vi "CFG Read_Write File.vi"(0 "Cluster In Ref":refnum<vi>, 1 "System Configuration File":path=path "inifiles/System Configuration.ini", 2 "Array In":T1[](array[typedef]), 5 "Cluster Out Ref":refnum<vi>, 7 "Enum Ref":refnum<vi>, 11 "Error In (no error)":errorcluster, 12 "Keys (Empty:All)":string[](array[string]), 13 "Operation":T5) -> (4 "Array":T1[](array[typedef]), 15 "Error Out":errorcluster)   [LabVIEW 2012]
uses:
  Type Defs/CFG File Operation Enum.ctl
  Type Defs/CFG Key Cluster.ctl
  Type Defs/CFG Tag Type Enum.ctl
  <vilib>/Utility/config.llb/Read Key (Boolean).vi
  <vilib>/Utility/config.llb/Read Key (String).vi
  <vilib>/Utility/config.llb/Read Key (Path).vi
  <vilib>/Utility/config.llb/Write Key (String).vi
  <vilib>/Utility/config.llb/Write Key (Boolean).vi
  <vilib>/Utility/config.llb/Write Key (Path).vi
  <vilib>/Utility/config.llb/NI_LVConfig.lvlib
panel:
  in  "Test Enum":T3(ring)
  in  "Test System In":T4 {"Settings"."Frequency" format="%_4p Hz"; "Settings"."Power" format="%.3f"; "Settings"."Code" format="%.0x"}
  out "Test System Out":T4 {"Settings"."Frequency" format="%_4p Hz"; "Settings"."Power" format="%.3f"; "Settings"."Code" format="%.0x"}
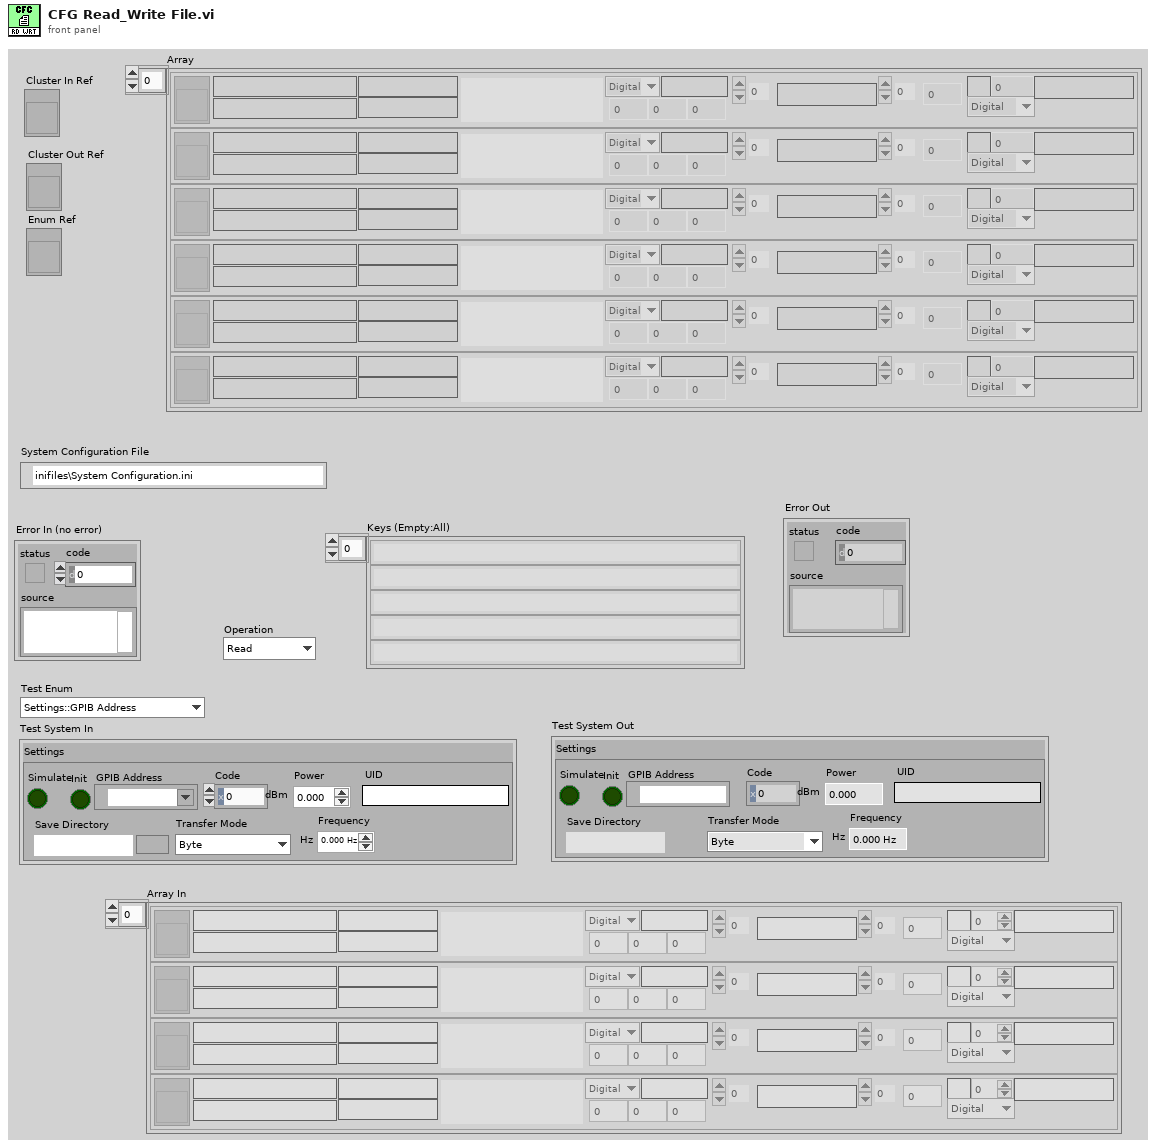
[diagram p1: front panel]
types:
  T1 = typedef "CFG Key Cluster.ctl" = cluster{"Strings []":string[], "Disabled Items []":i32[], "Value":variant, "Format String":string, "Tag":string, "Type":T2, "Section":string, " Ctl Ref":refnum<vi>, "Data Range":cluster{"Minimum":dbl, "Maximum":dbl, "Increment":dbl}, "Unit":string, "Special Instructions":string, "Delimiter(s)":string, "Dimensions":i32, "Element Type":T2, "Array Value String":string}
  T2 = typedef "CFG Tag Type Enum.ctl" = enum16{"Digital", "Slide", "Enum", "Boolean", "String", "Path", "Array", "VISAResourceName", "DAQmxName", "Cluster"}
  T3 = enum16{"Settings::GPIB Address", "Settings::Simulate", "Settings::Code", "Settings::Power", "Settings::UID", "Settings::Save Directory", "Settings::Transfer Mode", "Settings::Frequency"}
  T4 = cluster{"Settings":cluster{"Simulate":bool, "Init":bool, "GPIB Address":refnum<visa-resource-name>, "Save Directory":path, "Transfer Mode":enum16{"Byte", "Word", "LongWord"}, "Code":u8, "Power":dbl, "Frequency":dbl, "UID":string}}
  T5 = typedef "CFG File Operation Enum.ctl" = enum16{"Read", "Write", "Copy", "Edit"}
  T6 = typedef "NI_LVConfig.lvlib/Config Data RefNum.ctl" = refnum<k1>
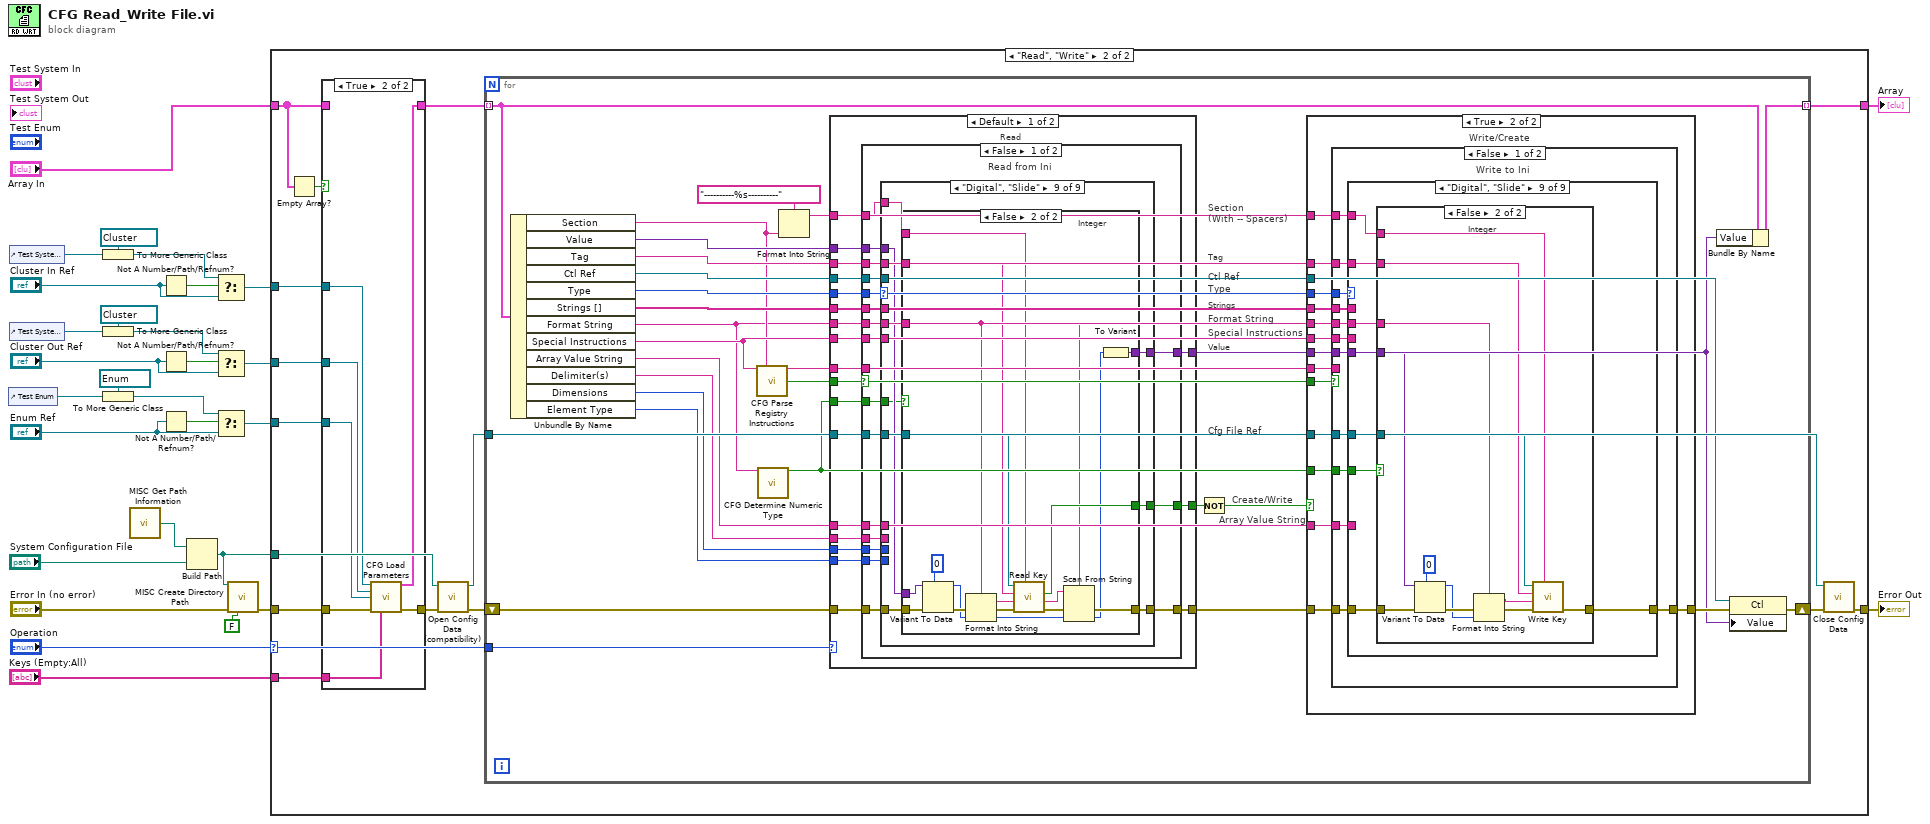
[diagram p0: block diagram]
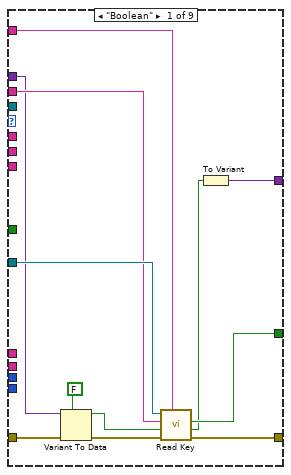
[diagram p4: hidden frame]
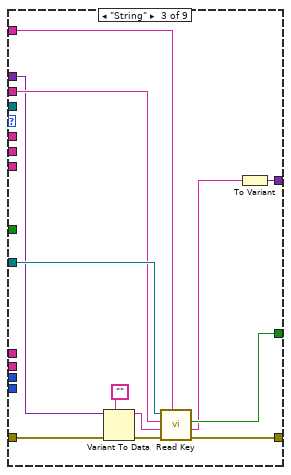
[diagram p6: hidden frame]
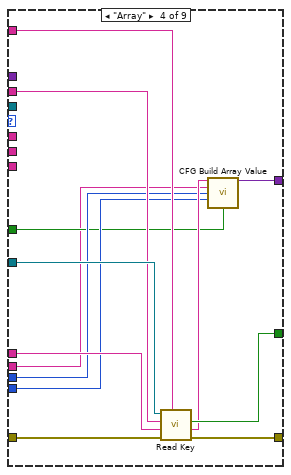
[diagram p7: hidden frame]
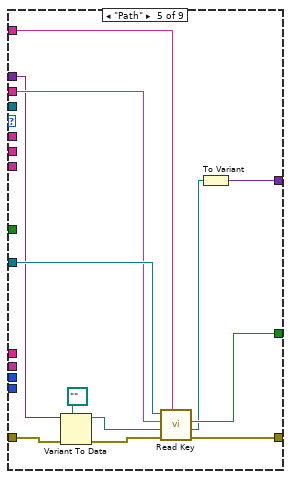
[diagram p8: hidden frame]
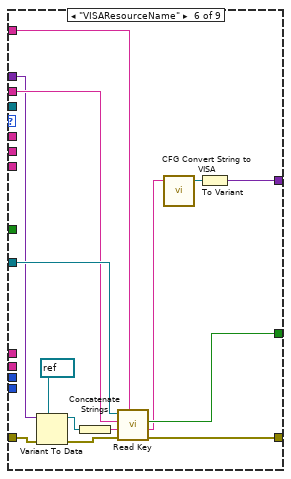
[diagram p9: hidden frame]
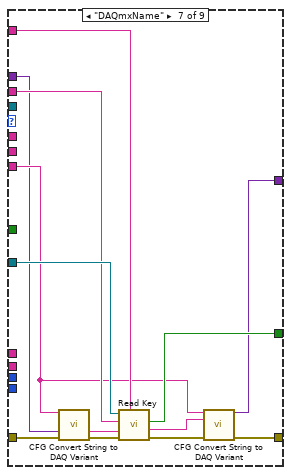
[diagram p10: hidden frame]
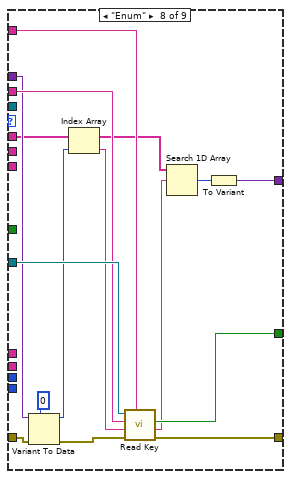
[diagram p11: hidden frame]
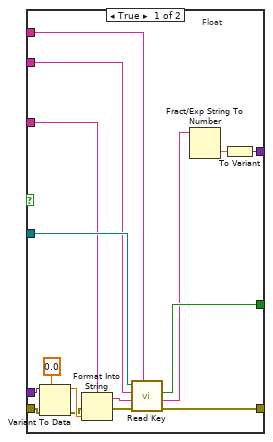
[diagram p12: hidden frame]
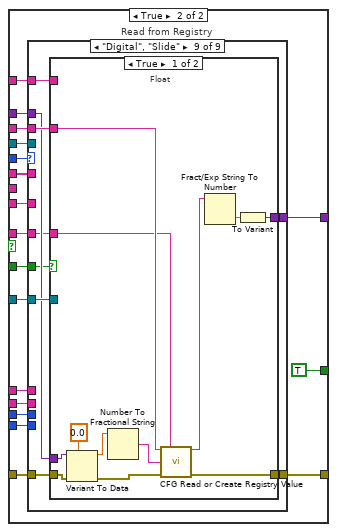
[diagram p13: hidden frame]
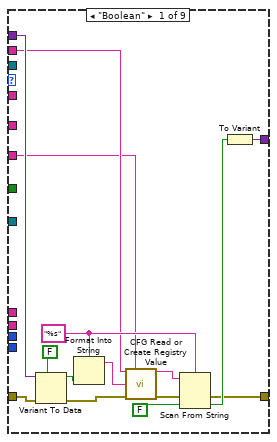
[diagram p14: hidden frame]
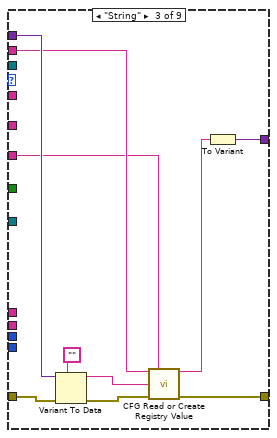
[diagram p16: hidden frame]
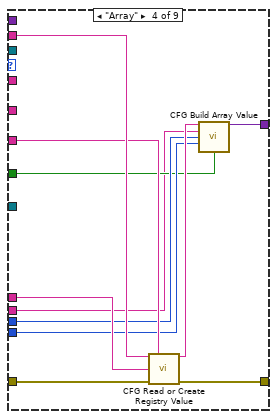
[diagram p17: hidden frame]
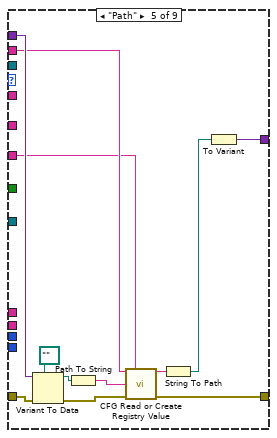
[diagram p18: hidden frame]
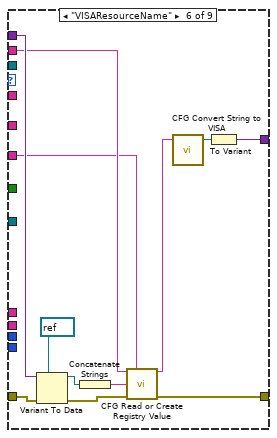
[diagram p19: hidden frame]
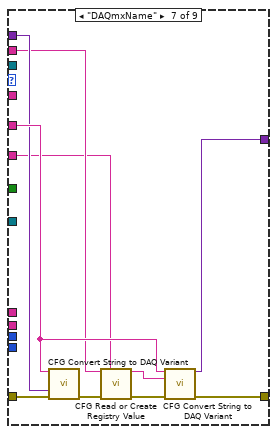
[diagram p20: hidden frame]
diagram:
  n1 = control-ref of="Test Enum"() -> (w2:refnum<vi>)
  n2 = control-ref of="Test System In"() -> (w21:refnum<vi>)
  n3 = control-ref of="Test System Out"() -> (w8:refnum<vi>)
  n4 = To More Generic Class(target class=refnum<vi> refnum ("Cluster Ref"), reference=w21) -> (generic class reference=w15:refnum<vi>)
  n5 = To More Generic Class(target class=refnum<vi> refnum ("Cluster Ref"), reference=w8) -> (generic class reference=w11:refnum<vi>)
  n6 = To More Generic Class(target class=refnum<vi> refnum ("Enum Ref"), reference=w2) -> (generic class reference=w5:refnum<vi>)
  n7 = call "MISC Get Path Information.vi"() -> ("Support Directory"=w24:path)  [unwired: 1 in, 14 out]
  n8 = Not A Number/Path/Refnum?(number/path/refnum="Cluster In Ref") -> (NaN/Path/Refnum?=w17:bool)
  n9 = Not A Number/Path/Refnum?(number/path/refnum="Cluster Out Ref") -> (NaN/Path/Refnum?=w10:bool)
  n10 = Not A Number/Path/Refnum?(number/path/refnum="Enum Ref") -> (NaN/Path/Refnum?=w13:bool)
  n11 = Build Path(base path=w24, name or relative path="System Configuration File") -> (appended path=w23:path)
  n12 = Select(t=w15, s=w17, f="Cluster In Ref") -> (s? t:f=w14:refnum<vi>)
  n13 = Select(t=w11, s=w10, f="Cluster Out Ref") -> (s? t:f=w6:refnum<vi>)
  n14 = Select(t=w5, s=w13, f="Enum Ref") -> (s? t:f=w1:refnum<vi>)
  n15 = call "MISC Create Directory Path.vi"("Path"=w23, "Error In (no error)"="Error In (no error)", "Input Type (T:Directories only)"=FALSE) -> ("Error Out"=w25:errorcluster)  [unwired: 12 out]
  n16 = case shown="\"Read\", \"Write\"" "Operation" {
    selector: "Operation" -> [_ w46]
    tunnel: w25 -> [w30 w40]
    tunnel: [w30 w44] -> w27
    tunnel: w23 -> [_ w42]
    tunnel: w14 -> [_ w38]
    tunnel: w1 -> [_ w36]
    tunnel: [_ w37] -> w18
    tunnel: w6 -> [_ w35]
    tunnel: "Keys (Empty:All)" -> [_ w34]
    tunnel: "Array In" -> [_ w33]
    frame Default {
    }
    frame "Read", "Write" {
      n17 = Empty Array?(array=w33) -> (empty?=w31:bool)
      n18 = case shown="True" w31 {
        tunnel: w40 -> [w47 w55]
        tunnel: [w47 w54] -> w39
        tunnel: w38 -> [_ w53]
        tunnel: w36 -> [_ w52]
        tunnel: w35 -> [_ w51]
        tunnel: w34 -> [_ w50]
        tunnel: w33 -> [w48 _]
        tunnel: [w48 w49] -> w32
        frame False {
        }
        frame True {
          n19 = call "CFG Load Parameters.vi"("Cluster In Ref"=w53, "Cluster Out Ref"=w51, "Enum Ref"=w52, "Error in (no error)"=w55, "Keys (Empty:All)"=w50) -> ("Param/Limits"=w49:T1[], "error out"=w54:errorcluster)  [unwired: 9 out]
        }
      }
      n20 = call <vilib>:"Open Config Data (compatibility).vi"("error in (no error)"=w39, "configuration file path"=w42) -> ("error out"=w43:errorcluster, "refnum"=w41:T6)  [unwired: 7 in, 1 out]
      n21 = for {
        tunnel: w41 -> [w79]
        shift-right: [w72] -> w45
        shift-left: w43 -> [w83]
        tunnel: w46 -> [w82]
        tunnel: w32 -> [w70] mode=indexing
        tunnel: [w69] -> w37 mode=indexing
        # "Array Value String"
        # "Special Instructions"
        # "Format String"
        # "Strings"
        # "Type"
        # "Ctl Ref"
        # "Tag"
        # "Section\n(With -- Spacers)"
        # "Value"
        # "Cfg File Ref"
        # "Create/Write"
        n22 = Unbundle By Name(w70) -> ("Section"=w63:string, "Value"=w77:variant, "Tag"=w76:string, "Ctl Ref"=w71:refnum<vi>, "Type"=w74:T2, "Strings []"=w75:string[], "Format String"=w60:string, "Special Instructions"=w64:string, "Array Value String"=w56:string, "Delimiter(s)"=w59:string, "Dimensions"=w58:i32, "Element Type"=w57:T2)
        n23 = call "CFG Parse Registry Instructions.vi"("Special Instructions"=w64, "Section"=w63) -> ("Subkey"=w61:string, "Registry Item"=w62:bool)  [unwired: 12 out]
        n24 = call "CFG Determine Numeric Type.vi"("Format String"=w60) -> ("Float"=w67:bool)  [unwired: 14 out]
        n25 = Format Into String(format string="----------%s----------", w63) -> (resulting string=w65:string)  [unwired: 2 in, 1 out]
        n26 = case shown="Default" w82 {
          tunnel: w83 -> [w103 w393]
          tunnel: [w102 w393] -> w80
          tunnel: w79 -> [w101 _]
          tunnel: w77 -> [w95 w392]
          tunnel: [w100 w392] -> w68
          tunnel: [w99 _] -> w81
          tunnel: w65 -> [w98 _]
          tunnel: w76 -> [w97 _]
          tunnel: w74 -> [w96 _]
          tunnel: w75 -> [w94 _]
          tunnel: w71 -> [w93 _]
          tunnel: w67 -> [w92 _]
          tunnel: w64 -> [w91 _]
          tunnel: w62 -> [w90 _]
          tunnel: w61 -> [w89 _]
          tunnel: w60 -> [w88 _]
          tunnel: w56 -> [w87 _]
          tunnel: w59 -> [w86 _]
          tunnel: w58 -> [w85 _]
          tunnel: w57 -> [w84 _]
          frame Default {
            # "Read"
            n27 = case shown="False" w90 {
              tunnel: w103 -> [w121 w274]
              tunnel: [w120 w273] -> w102
              tunnel: w101 -> [w119 w272]
              tunnel: [w118 w271] -> w100
              tunnel: [w117 TRUE ("found?")] -> w99
              tunnel: w98 -> [w116 w270]
              tunnel: w97 -> [w115 w269]
              tunnel: w96 -> [w114 w268]
              tunnel: w95 -> [w113 w267]
              tunnel: w94 -> [w112 w266]
              tunnel: w93 -> [w111 w265]
              tunnel: w92 -> [w110 w264]
              tunnel: w91 -> [w109 w263]
              tunnel: w89 -> [_ w262]
              tunnel: w88 -> [w108 _]
              tunnel: w87 -> [w107 w260]
              tunnel: w86 -> [w106 w257]
              tunnel: w85 -> [w105 w259]
              tunnel: w84 -> [w104 w258]
              frame False {
                # "Read from Ini"
                n28 = case shown="\"Digital\", \"Slide\"" w114 {
                  tunnel: w121 -> [w126 w134 w140 w147 w164 w180 w189 w207 w217]
                  tunnel: [w133 w134 w146 w159 w171 w185 w191 w213 w223] -> w120
                  tunnel: w119 -> [w132 _ w145 w158 w170 w184 w198 w212 w222]
                  tunnel: [w127 _ w141 w152 w165 w173 w193 w208 w218] -> w118
                  tunnel: [w131 _ w144 w157 w169 w183 w197 w211 w221] -> w117
                  tunnel: w116 -> [w130 _ w138 w155 w168 w182 w196 w210 w220]
                  tunnel: w115 -> [w129 _ w143 w156 w167 w181 w195 w209 w219]
                  tunnel: w113 -> [w124 _ w139 _ w162 w178 w188 w204 w216]
                  tunnel: w112 -> [_ _ _ _ _ _ _ w201 _]
                  tunnel: w111 -> [_ _ _ _ _ _ _ _ _]
                  tunnel: w110 -> [_ _ _ w149 _ _ _ _ w215]
                  tunnel: w109 -> [_ _ _ _ _ _ w190 _ _]
                  tunnel: w108 -> [_ _ _ _ _ _ _ _ w214]
                  tunnel: w107 -> [_ _ _ w154 _ _ _ _ _]
                  tunnel: w106 -> [_ _ _ w148 _ _ _ _ _]
                  tunnel: w105 -> [_ _ _ w151 _ _ _ _ _]
                  tunnel: w104 -> [_ _ _ w150 _ _ _ _ _]
                  frame "Boolean" {
                    n29 = Variant To Data(error in=w126, type=FALSE ("default value"), Variant=w124) -> (data=w122:bool, error out=w125:errorcluster)
                    n30 = call-poly <vilib>:"Read Key.vi"("section"=w130, "error in (no error)"=w125, "default value"=w122, "key"=w129, "refnum"=w132) -> ("error out"=w133:errorcluster, "value"=w128:bool, "found?"=w131:bool)  [unwired: 4 out]
                    n31 = To Variant(anything=w128) -> (Variant=w127:variant)
                  }
                  frame "Cluster" {
                  }
                  frame "String" {
                    n32 = Variant To Data(error in=w140, type="", Variant=w139) -> (data=w136:string, error out=w137:errorcluster)
                    n33 = call-poly <vilib>:"Read Key.vi"("section"=w138, "error in (no error)"=w137, "default value"=w136, "key"=w143, "refnum"=w145) -> ("error out"=w146:errorcluster, "value"=w142:string, "found?"=w144:bool)  [unwired: 1 in, 3 out]
                    n34 = To Variant(anything=w142) -> (Variant=w141:variant)
                  }
                  frame "Array" {
                    n35 = call-poly <vilib>:"Read Key.vi"("section"=w155, "error in (no error)"=w147, "default value"=w154, "key"=w156, "refnum"=w158) -> ("error out"=w159:errorcluster, "value"=w153:string, "found?"=w157:bool)  [unwired: 1 in, 3 out]
                    n36 = call "CFG Build Array Value.vi"("Value String"=w153, "Delimiter(s)"=w148, "Dimensions"=w151, "Element Type"=w150, "Float"=w149) -> ("Variant"=w152:variant)  [unwired: 1 in, 9 out]
                  }
                  frame "Path" {
                    n37 = Variant To Data(error in=w164, type=path "", Variant=w162) -> (data=w161:path, error out=w163:errorcluster)
                    n38 = call-poly <vilib>:"Read Key.vi"("section"=w168, "error in (no error)"=w163, "default value"=w161, "key"=w167, "refnum"=w170) -> ("error out"=w171:errorcluster, "value"=w166:path, "found?"=w169:bool)  [unwired: 4 out]
                    n39 = To Variant(anything=w166) -> (Variant=w165:variant)
                  }
                  frame "VISAResourceName" {
                    n40 = Variant To Data(error in=w180, type=refnum<visa-resource-name> refnum ("GPIB Address"), Variant=w178) -> (data=w177:refnum<visa-resource-name>, error out=w179:errorcluster)
                    n41 = Concatenate Strings(w177) -> (w176:string)
                    n42 = call-poly <vilib>:"Read Key.vi"("section"=w182, "error in (no error)"=w179, "default value"=w176, "key"=w181, "refnum"=w184) -> ("error out"=w185:errorcluster, "value"=w174:string, "found?"=w183:bool)  [unwired: 1 in, 3 out]
                    n43 = call "CFG Convert String to VISA.vi"("VISA String"=w174) -> ("VISA Resource"=w172:refnum<visa-resource-name>)  [unwired: 4 out]
                    n44 = To Variant(anything=w172) -> (Variant=w173:variant)
                  }
                  frame "DAQmxName" {
                    n45 = call "CFG Convert String to DAQ Variant.vi"("Special Instructions"=w190, "Value Variant In"=w188, "error in"=w189) -> ("Value String Out"=w187:string, "error out"=w186:errorcluster)  [unwired: 1 in, 10 out]
                    n46 = call-poly <vilib>:"Read Key.vi"("section"=w196, "error in (no error)"=w186, "default value"=w187, "key"=w195, "refnum"=w198) -> ("error out"=w192:errorcluster, "value"=w194:string, "found?"=w197:bool)  [unwired: 1 in, 3 out]
                    n47 = call "CFG Convert String to DAQ Variant.vi"("Special Instructions"=w190, "Value String in"=w194, "error in"=w192) -> ("Value Variant Out"=w193:variant, "error out"=w191:errorcluster)  [unwired: 1 in, 10 out]
                  }
                  frame "Enum" {
                    n48 = Variant To Data(error in=w207, type=0, Variant=w204) -> (data=w203:i32, error out=w206:errorcluster)
                    n49 = Index Array(array=w201, index=w203) -> (element=w202:string)
                    n50 = call-poly <vilib>:"Read Key.vi"("section"=w210, "error in (no error)"=w206, "default value"=w202, "key"=w209, "refnum"=w212) -> ("error out"=w213:errorcluster, "value"=w200:string, "found?"=w211:bool)  [unwired: 1 in, 3 out]
                    n51 = Search 1D Array(1D array=w201, element=w200) -> (index of element=w199:i32)  [unwired: 1 out]
                    n52 = To Variant(anything=w199) -> (Variant=w208:variant)
                  }
                  frame "Digital", "Slide" {
                    n53 = case shown="False" w215 {
                      tunnel: [w226 w244] -> w223
                      tunnel: w222 -> [w239 w256]
                      tunnel: [w238 w255] -> w221
                      tunnel: w220 -> [w237 w254]
                      tunnel: w219 -> [w236 w253]
                      tunnel: w217 -> [w232 w249]
                      tunnel: w216 -> [w233 w250]
                      tunnel: [w235 w252] -> w218
                      tunnel: w214 -> [w227 w243]
                      frame True {
                        # "Float"
                        n54 = Variant To Data(error in=w232, type=0.0, Variant=w233) -> (data=w231:dbl, error out=w230:errorcluster)
                        n55 = Format Into String(format string=w227, error in=w230, w231) -> (resulting string=w228:string, error out=w229:errorcluster)  [unwired: 1 in]
                        n56 = call-poly <vilib>:"Read Key.vi"("section"=w237, "error in (no error)"=w229, "default value"=w228, "key"=w236, "refnum"=w239) -> ("error out"=w226:errorcluster, "value"=w225:string, "found?"=w238:bool)  [unwired: 1 in, 3 out]
                        n57 = Fract/Exp String To Number(string=w225) -> (number=w224:dbl)  [unwired: 3 in, 1 out]
                        n58 = To Variant(anything=w224) -> (Variant=w235:variant)
                      }
                      frame False {
                        # "Integer"
                        n59 = Variant To Data(error in=w249, type=0, Variant=w250) -> (data=w240:i32, error out=w248:errorcluster)
                        n60 = Format Into String(format string=w243, error in=w248, w240) -> (resulting string=w246:string, error out=w247:errorcluster)  [unwired: 1 in]
                        n61 = call-poly <vilib>:"Read Key.vi"("section"=w254, "error in (no error)"=w247, "default value"=w246, "key"=w253, "refnum"=w256) -> ("error out"=w245:errorcluster, "value"=w242:string, "found?"=w255:bool)  [unwired: 1 in, 3 out]
                        n62 = Scan From String(format string=w243, input string=w242, error in=w245, default 1=w240) -> (error out=w244:errorcluster, output 1=w241:i32)  [unwired: 1 in, 2 out]
                        n63 = To Variant(anything=w241) -> (Variant=w252:variant)
                      }
                    }
                  }
                }
              }
              frame True {
                # "Read from Registry"
                n64 = case shown="\"Digital\", \"Slide\"" w268 {
                  tunnel: w274 -> [w288 w290 w299 w307 w322 w335 w342 w357 w362]
                  tunnel: [w275 w290 w295 w311 w315 w328 w344 w350 w367] -> w273
                  tunnel: w272 -> [_ _ _ _ _ _ _ _ w366]
                  tunnel: [w289 _ w300 w305 w323 w331 w345 w358 w363] -> w271
                  tunnel: w270 -> [_ _ _ _ _ _ _ _ w365]
                  tunnel: w269 -> [w278 _ w293 w310 w317 w325 w337 w348 w364]
                  tunnel: w267 -> [w287 _ w298 _ w321 w334 w341 w355 w361]
                  tunnel: w266 -> [_ _ _ _ _ _ _ w353 _]
                  tunnel: w265 -> [_ _ _ _ _ _ _ _ _]
                  tunnel: w264 -> [_ _ _ w302 _ _ _ _ w360]
                  tunnel: w263 -> [_ _ _ _ _ _ w343 _ _]
                  tunnel: w262 -> [w277 _ w291 w309 w312 w324 w336 w346 w359]
                  tunnel: w260 -> [_ _ _ w308 _ _ _ _ _]
                  tunnel: w259 -> [_ _ _ w304 _ _ _ _ _]
                  tunnel: w258 -> [_ _ _ w303 _ _ _ _ _]
                  tunnel: w257 -> [_ _ _ w301 _ _ _ _ _]
                  frame "Boolean" {
                    w281 = "%s" ("format string")
                    n65 = Variant To Data(error in=w288, type=FALSE ("default value"), Variant=w287) -> (data=w284:bool, error out=w285:errorcluster)
                    n66 = Format Into String(format string=w281, w284) -> (resulting string=w283:string)  [unwired: 2 in, 1 out]
                    n67 = call "CFG Read or Create Registry Value.vi"("Tag (Value)"=w278, "Subkey"=w277, "Default (Data)"=w283, "error in (no error)"=w285) -> ("Data"=w282:string, "error out"=w276:errorcluster)  [unwired: 10 out]
                    n68 = Scan From String(format string=w281, input string=w282, error in=w276, default 1=FALSE ("default value")) -> (error out=w275:errorcluster, output 1=w279:bool)  [unwired: 1 in, 2 out]
                    n69 = To Variant(anything=w279) -> (Variant=w289:variant)
                  }
                  frame "Cluster" {
                  }
                  frame "String" {
                    n70 = Variant To Data(error in=w299, type="", Variant=w298) -> (data=w292:string, error out=w296:errorcluster)
                    n71 = call "CFG Read or Create Registry Value.vi"("Tag (Value)"=w293, "Subkey"=w291, "Default (Data)"=w292, "error in (no error)"=w296) -> ("Data"=w294:string, "error out"=w295:errorcluster)  [unwired: 10 out]
                    n72 = To Variant(anything=w294) -> (Variant=w300:variant)
                  }
                  frame "Array" {
                    n73 = call "CFG Read or Create Registry Value.vi"("Tag (Value)"=w310, "Subkey"=w309, "Default (Data)"=w308, "error in (no error)"=w307) -> ("Data"=w306:string, "error out"=w311:errorcluster)  [unwired: 10 out]
                    n74 = call "CFG Build Array Value.vi"("Value String"=w306, "Delimiter(s)"=w301, "Dimensions"=w304, "Element Type"=w303, "Float"=w302) -> ("Variant"=w305:variant)  [unwired: 1 in, 9 out]
                  }
                  frame "Path" {
                    n75 = Variant To Data(error in=w322, type=path "", Variant=w321) -> (data=w319:path, error out=w316:errorcluster)
                    n76 = Path To String(path=w319) -> (string=w318:string)
                    n77 = call "CFG Read or Create Registry Value.vi"("Tag (Value)"=w317, "Subkey"=w312, "Default (Data)"=w318, "error in (no error)"=w316) -> ("Data"=w314:string, "error out"=w315:errorcluster)  [unwired: 10 out]
                    n78 = String To Path(string=w314) -> (path=w313:path)
                    n79 = To Variant(anything=w313) -> (Variant=w323:variant)
                  }
                  frame "VISAResourceName" {
                    n80 = Variant To Data(error in=w335, type=refnum<visa-resource-name> refnum ("GPIB Address"), Variant=w334) -> (data=w333:refnum<visa-resource-name>, error out=w329:errorcluster)
                    n81 = Concatenate Strings(w333) -> (w326:string)
                    n82 = call "CFG Read or Create Registry Value.vi"("Tag (Value)"=w325, "Subkey"=w324, "Default (Data)"=w326, "error in (no error)"=w329) -> ("Data"=w327:string, "error out"=w328:errorcluster)  [unwired: 10 out]
                    n83 = call "CFG Convert String to VISA.vi"("VISA String"=w327) -> ("VISA Resource"=w330:refnum<visa-resource-name>)  [unwired: 4 out]
                    n84 = To Variant(anything=w330) -> (Variant=w331:variant)
                  }
                  frame "DAQmxName" {
                    n85 = call "CFG Convert String to DAQ Variant.vi"("Special Instructions"=w343, "Value Variant In"=w341, "error in"=w342) -> ("error out"=w340:errorcluster)  [unwired: 1 in, 11 out]
                    n86 = call "CFG Read or Create Registry Value.vi"("Tag (Value)"=w337, "Subkey"=w336, "error in (no error)"=w340) -> ("Data"=w338:string, "error out"=w339:errorcluster)  [unwired: 1 in, 10 out]
                    n87 = call "CFG Convert String to DAQ Variant.vi"("Special Instructions"=w343, "Value String in"=w338, "error in"=w339) -> ("Value Variant Out"=w345:variant, "error out"=w344:errorcluster)  [unwired: 1 in, 10 out]
                  }
                  frame "Enum" {
                    n88 = Variant To Data(error in=w357, type=0, Variant=w355) -> (data=w354:i32, error out=w351:errorcluster)
                    n89 = Index Array(array=w353, index=w354) -> (element=w347:string)
                    n90 = call "CFG Read or Create Registry Value.vi"("Tag (Value)"=w348, "Subkey"=w346, "Default (Data)"=w347, "error in (no error)"=w351) -> ("Data"=w349:string, "error out"=w350:errorcluster)  [unwired: 10 out]
                    n91 = Search 1D Array(1D array=w353, element=w349) -> (index of element=w352:i32)  [unwired: 1 out]
                    n92 = To Variant(anything=w352) -> (Variant=w358:variant)
                  }
                  frame "Digital", "Slide" {
                    n93 = case shown="True" w360 {
                      tunnel: [w371 w383] -> w367
                      tunnel: w366 -> [_ _]
                      tunnel: w365 -> [_ _]
                      tunnel: w364 -> [w370 w382]
                      tunnel: w362 -> [w376 w388]
                      tunnel: w361 -> [w377 w389]
                      tunnel: [w379 w391] -> w363
                      tunnel: w359 -> [w369 w381]
                      frame True {
                        # "Float"
                        n94 = Variant To Data(error in=w376, type=0.0, Variant=w377) -> (data=w375:dbl, error out=w373:errorcluster)
                        n95 = Number To Fractional String(number=w375) -> (F-format string=w372:string)  [unwired: 3 out]
                        n96 = call "CFG Read or Create Registry Value.vi"("Tag (Value)"=w370, "Subkey"=w369, "Default (Data)"=w372, "error in (no error)"=w373) -> ("Data"=w368:string, "error out"=w371:errorcluster)  [unwired: 10 out]
                        n97 = Fract/Exp String To Number(string=w368) -> (number=w374:dbl)  [unwired: 4 out]
                        n98 = To Variant(anything=w374) -> (Variant=w379:variant)
                      }
                      frame False {
                        # "Integer"
                        n99 = Variant To Data(error in=w388, type=0, Variant=w389) -> (data=w387:i32, error out=w385:errorcluster)
                        n100 = Number To Decimal String(number=w387) -> (decimal integer string=w384:string)  [unwired: 1 out]
                        n101 = call "CFG Read or Create Registry Value.vi"("Tag (Value)"=w382, "Subkey"=w381, "Default (Data)"=w384, "error in (no error)"=w385) -> ("Data"=w380:string, "error out"=w383:errorcluster)  [unwired: 10 out]
                        n102 = Decimal String To Number(string=w380) -> (number=w386:i32)  [unwired: 3 out]
                        n103 = To Variant(anything=w386) -> (Variant=w391:variant)
                      }
                    }
                  }
                }
              }
            }
          }
          frame "Write" {
            # "No Read"
          }
        }
        n104 = Not(x=w81) -> (.not. x?=w78:bool)
        n105 = case shown="True" w78 {
          tunnel: w80 -> [w394 w403]
          tunnel: [w394 w408] -> w73
          tunnel: w79 -> [_ w407]
          tunnel: w76 -> [_ w406]
          tunnel: w68 -> [_ w404]
          tunnel: w65 -> [_ w405]
          tunnel: w71 -> [_ _]
          tunnel: w75 -> [_ w401]
          tunnel: w60 -> [_ w396]
          tunnel: w74 -> [_ w402]
          tunnel: w67 -> [_ w400]
          tunnel: w64 -> [_ w399]
          tunnel: w62 -> [_ w398]
          tunnel: w61 -> [_ w397]
          tunnel: w56 -> [_ w395]
          frame False {
            # "Key Found/No Write"
          }
          frame True {
            # "Write/Create"
            n106 = case shown="False" w398 {
              tunnel: [w420 w520] -> w408
              tunnel: w407 -> [w419 w528]
              tunnel: w406 -> [w418 w518]
              tunnel: w405 -> [w417 _]
              tunnel: w404 -> [w416 w527]
              tunnel: w403 -> [w415 w526]
              tunnel: w402 -> [w414 w525]
              tunnel: w401 -> [w413 w524]
              tunnel: w400 -> [w412 w523]
              tunnel: w399 -> [w411 w522]
              tunnel: w397 -> [_ w519]
              tunnel: w396 -> [w410 _]
              tunnel: w395 -> [w409 w516]
              frame False {
                # "Write to Ini"
                n107 = case shown="\"Digital\", \"Slide\"" w414 {
                  tunnel: [w431 w432 w441 w450 w456 w465 w474 w483 w491] -> w420
                  tunnel: w419 -> [w430 _ w440 w449 w455 w464 w473 w482 w490]
                  tunnel: w418 -> [w429 _ w439 w448 w454 w463 w472 w481 w489]
                  tunnel: w417 -> [w428 _ w433 w447 w453 w462 w471 w480 w488]
                  tunnel: w416 -> [w423 _ w436 w444 _ w459 w468 w476 w486]
                  tunnel: w415 -> [w425 w432 w438 w446 w451 w461 w470 w478 w487]
                  tunnel: w413 -> [w422 _ _ _ _ _ _ _ _]
                  tunnel: w412 -> [_ _ _ _ _ _ _ _ w485]
                  tunnel: w411 -> [_ _ _ _ _ _ _ w479 _]
                  tunnel: w410 -> [_ _ _ _ _ _ _ _ w484]
                  tunnel: w409 -> [_ _ _ _ w452 _ _ _ _]
                  frame "Enum" {
                    n108 = Variant To Data(error in=w425, type=0, Variant=w423) -> (data=w427:i32, error out=w424:errorcluster)
                    n109 = Index Array(array=w422, index=w427) -> (element=w421:string)
                    n110 = call-poly <vilib>:"Write Key.vi"("section"=w428, "error in (no error)"=w424, "value"=w421, "key"=w429, "refnum"=w430) -> ("error out"=w431:errorcluster)  [unwired: 1 in, 5 out]
                  }
                  frame "Cluster" {
                  }
                  frame "Boolean" {
                    n111 = Variant To Data(error in=w438, type=FALSE ("default value"), Variant=w436) -> (data=w434:bool, error out=w437:errorcluster)
                    n112 = call-poly <vilib>:"Write Key.vi"("section"=w433, "error in (no error)"=w437, "value"=w434, "key"=w439, "refnum"=w440) -> ("error out"=w441:errorcluster)  [unwired: 6 out]
                  }
                  frame "String" {
                    n113 = Variant To Data(error in=w446, type="", Variant=w444) -> (data=w443:string, error out=w445:errorcluster)
                    n114 = call-poly <vilib>:"Write Key.vi"("section"=w447, "error in (no error)"=w445, "value"=w443, "key"=w448, "refnum"=w449) -> ("error out"=w450:errorcluster)  [unwired: 1 in, 5 out]
                  }
                  frame "Array" {
                    n115 = call-poly <vilib>:"Write Key.vi"("section"=w453, "error in (no error)"=w451, "value"=w452, "key"=w454, "refnum"=w455) -> ("error out"=w456:errorcluster)  [unwired: 1 in, 5 out]
                  }
                  frame "Path" {
                    n116 = Variant To Data(error in=w461, type=path "", Variant=w459) -> (data=w458:path, error out=w460:errorcluster)
                    n117 = call-poly <vilib>:"Write Key.vi"("section"=w462, "error in (no error)"=w460, "value"=w458, "key"=w463, "refnum"=w464) -> ("error out"=w465:errorcluster)  [unwired: 6 out]
                  }
                  frame "VISAResourceName" {
                    n118 = Variant To Data(error in=w470, type="", Variant=w468) -> (data=w467:string, error out=w469:errorcluster)
                    n119 = call-poly <vilib>:"Write Key.vi"("section"=w471, "error in (no error)"=w469, "value"=w467, "key"=w472, "refnum"=w473) -> ("error out"=w474:errorcluster)  [unwired: 1 in, 5 out]
                  }
                  frame "DAQmxName" {
                    n120 = call "CFG Convert String to DAQ Variant.vi"("Special Instructions"=w479, "Value Variant In"=w476, "error in"=w478) -> ("Value String Out"=w477:string, "error out"=w475:errorcluster)  [unwired: 1 in, 10 out]
                    n121 = call-poly <vilib>:"Write Key.vi"("section"=w480, "error in (no error)"=w475, "value"=w477, "key"=w481, "refnum"=w482) -> ("error out"=w483:errorcluster)  [unwired: 1 in, 5 out]
                  }
                  frame "Digital", "Slide" {
                    n122 = case shown="False" w485 {
                      tunnel: [w503 w515] -> w491
                      tunnel: w490 -> [w502 w514]
                      tunnel: w489 -> [w501 w513]
                      tunnel: w488 -> [w500 w512]
                      tunnel: w487 -> [w499 w511]
                      tunnel: w486 -> [w498 w510]
                      tunnel: w484 -> [w493 w504]
                      frame True {
                        # "Float"
                        n123 = Variant To Data(error in=w499, type=0.0, Variant=w498) -> (data=w494:dbl, error out=w496:errorcluster)
                        n124 = Format Into String(format string=w493, error in=w496, w494) -> (resulting string=w492:string, error out=w495:errorcluster)  [unwired: 1 in]
                        n125 = call-poly <vilib>:"Write Key.vi"("section"=w500, "error in (no error)"=w495, "value"=w492, "key"=w501, "refnum"=w502) -> ("error out"=w503:errorcluster)  [unwired: 1 in, 5 out]
                      }
                      frame False {
                        # "Integer"
                        n126 = Variant To Data(error in=w511, type=0, Variant=w510) -> (data=w506:i32, error out=w508:errorcluster)
                        n127 = Format Into String(format string=w504, error in=w508, w506) -> (resulting string=w505:string, error out=w507:errorcluster)  [unwired: 1 in]
                        n128 = call-poly <vilib>:"Write Key.vi"("section"=w512, "error in (no error)"=w507, "value"=w505, "key"=w513, "refnum"=w514) -> ("error out"=w515:errorcluster)  [unwired: 1 in, 5 out]
                      }
                    }
                  }
                }
              }
              frame True {
                # "Write to Registry"
                n129 = case shown="\"Digital\", \"Slide\"" w525 {
                  tunnel: [w529 w536 w539 w544 w549 w551 w557 w562 w568] -> w521
                  tunnel: w528 -> [_ _ _ _ _ _ _ _ w572]
                  tunnel: w527 -> [w532 _ w542 w547 _ w555 w560 w564 w570]
                  tunnel: w526 -> [w533 w536 w543 w548 w549 w556 w561 w565 w571]
                  tunnel: w524 -> [w531 _ _ _ _ _ _ _ _]
                  tunnel: w523 -> [_ _ _ _ _ _ _ _ w569]
                  tunnel: w522 -> [_ _ _ _ _ _ _ w566 _]
                  tunnel: [w530 _ w537 w545 w550 w552 w558 w563 w567] -> w517
                  tunnel: w516 -> [_ _ _ _ w550 _ _ _ _]
                  frame "Enum" {
                    n130 = Variant To Data(error in=w533, type=0, Variant=w532) -> (data=w535:i32, error out=w529:errorcluster)
                    n131 = Index Array(array=w531, index=w535) -> (element=w530:string)
                  }
                  frame "Cluster" {
                  }
                  frame "Boolean" {
                    n132 = Variant To Data(error in=w543, type=FALSE ("default value"), Variant=w542) -> (data=w538:bool, error out=w539:errorcluster)
                    n133 = Format Into String(format string="%s", w538) -> (resulting string=w537:string)  [unwired: 2 in, 1 out]
                  }
                  frame "String" {
                    n134 = Variant To Data(error in=w548, type="", Variant=w547) -> (data=w545:string, error out=w544:errorcluster)
                  }
                  frame "Array" {
                  }
                  frame "Path" {
                    n135 = Variant To Data(error in=w556, type=path "", Variant=w555) -> (data=w553:path, error out=w551:errorcluster)
                    n136 = Path To String(path=w553) -> (string=w552:string)
                  }
                  frame "VISAResourceName" {
                    n137 = Variant To Data(error in=w561, type="", Variant=w560) -> (data=w558:string, error out=w557:errorcluster)
                  }
                  frame "DAQmxName" {
                    n138 = call "CFG Convert String to DAQ Variant.vi"("Special Instructions"=w566, "Value Variant In"=w564, "error in"=w565) -> ("Value String Out"=w563:string, "error out"=w562:errorcluster)  [unwired: 1 in, 10 out]
                  }
                  frame "Digital", "Slide" {
                    n139 = case shown="True" w569 {
                      tunnel: [w573 w579] -> w568
                      tunnel: w572 -> [_ _]
                      tunnel: w571 -> [w578 w584]
                      tunnel: w570 -> [w577 w583]
                      tunnel: [w574 w580] -> w567
                      frame True {
                        # "Float"
                        n140 = Variant To Data(error in=w578, type=0.0, Variant=w577) -> (data=w575:dbl, error out=w573:errorcluster)
                        n141 = Number To Fractional String(number=w575) -> (F-format string=w574:string)  [unwired: 3 out]
                      }
                      frame False {
                        # "Integer"
                        n142 = Variant To Data(error in=w584, type=0, Variant=w583) -> (data=w581:i32, error out=w579:errorcluster)
                        n143 = Number To Decimal String(number=w581) -> (decimal integer string=w580:string)  [unwired: 1 out]
                      }
                    }
                  }
                }
                n144 = call "CFG Write Registry Value.vi"("Tag (Value)"=w518, "Subkey"=w519, "Data"=w517, "error in (no error)"=w521) -> ("error out"=w520:errorcluster)  [unwired: 11 out]
              }
            }
          }
        }
        n145 = Bundle By Name(cluster=w70, "Value"=w68) -> (w69:T1)
        n146 = property class="Ctl"(reference=w71, error in=w73, "Value"=w68) -> (error out=w72:errorcluster)  [unwired: 1 out]
      }
      n147 = call <vilib>:"Close Config Data.vi"("error in (no error)"=w45, "refnum"=w41) -> ("error out"=w44:errorcluster)  [unwired: 1 in, 8 out]
    }
  }
  "Error Out" <- w27
  "Array" <- w18
